vi "WaveformClientSide.vi"() -> ()   [LabVIEW 2019]
panel:
  out "Waveform Chart":dbl(graph)
  in  "stop wave from Client Side":bool
  out "error out":errorcluster
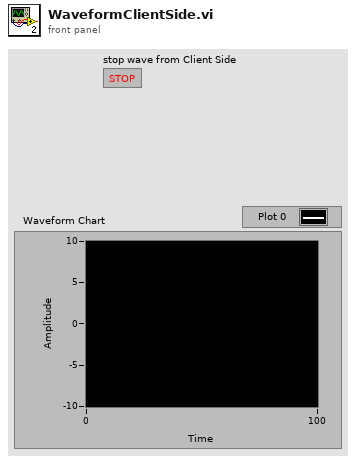
[diagram p1: front panel]
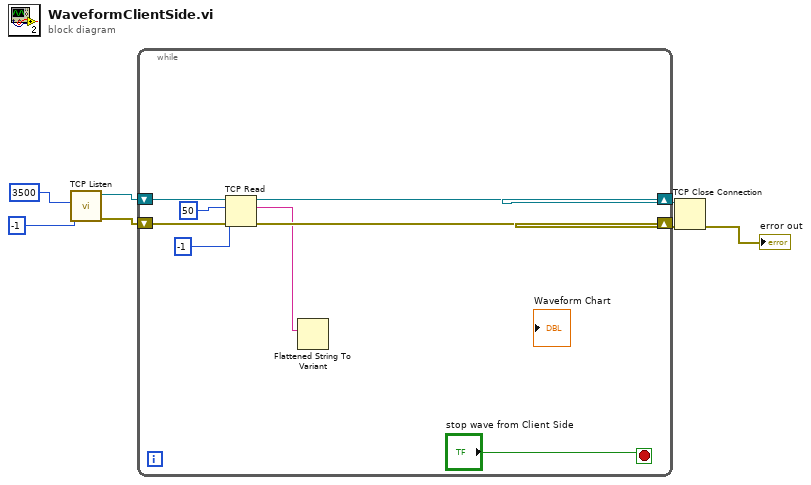
[diagram p0: block diagram]
diagram:
  n1 = call <vilib>:"TCP Listen.vi"("timeout ms (wait forever: -1)"=-1, "port"=u16 3500) -> ("error out"=w3:errorcluster, "connection ID"=w5:refnum<k5>)  [unwired: 5 in, 3 out]
  n2 = while {
    shift-right: [w14] -> w4
    shift-left: w5 -> [w15]
    shift-right: [w12] -> w2
    shift-left: w3 -> [w13]
    stop <- "stop wave from Client Side" stop-if-true
    n3 = TCP Read(connection ID=w15, bytes to read=50, error in (no error)=w13, 9:-1 ("timeout ms (25000)")) -> (connection ID out=w14:refnum<k5>, data out=w8:string, error out=w12:errorcluster)  [unwired: 1 in]
    n4 = Flattened String To Variant(6:w8) -> ()  [unwired: 2 in, 2 out]
  }
  n5 = TCP Close Connection(connection ID=w4, error in (no error)=w2) -> (error out=→"error out":errorcluster)  [unwired: 1 in, 1 out]
